vi "pco.labview_Live_Example_PSEUDO_COL.vi"() -> ()   [LabVIEW 2020]
doc: "A short program to demonstrate the fundamentals of control and image acquision with the pco.camera series. The program records a sequence of images, with \"live\" updating, until the \"StopRecording\" button is pressed. Use ctrl-H for more help on the individual controls and indicators.\n\nCopyright 2004, 2010 The Cooke Corporation."
uses:
  CameraAccess.lvlib
  ImageSensor.lvlib
  TimingControl.lvlib
  Recorder.lvlib
  RecordingControl.lvlib
  CameraDescription.lvlib
  Convert.lvlib
  GeneralCameraControl.lvlib
panel:
  in  "Auto Range Peak":bool
  in  "Auto Range Crop":bool
  in  "Load LUT":path
  in  "Gamma":dbl=1.0 min=0.009999999776482582 max=10.0 step=0.009999999776482582 format="%.2f"
  in  "iContrast [%]":i32 min=-100 max=100 step=1
  out "wImgBuf":u16[][](array[numeric])
  in  "Zoom [%]":i32(c297)=26
  in  "iScale_max":i32=2000 min=0 max=65535 step=1
  in  "iScale_min":i32=200 min=0 max=65535 step=1
  out "phConv":u64
  out "Image":picture
  out "Recorded Images":u32
  in  "TriggerMode":u16(ring) items=["auto sequence"=0, "software trigger"=1, "external exposure start & software trigger"=2, "external exposure control"=3, "external synchronized"=4, "fast external exposure control"=5, "external CDS control"=6, "slow external exposure control"=7, "external synchronized HDSDI"=258]
  in  "Quit":bool
  out "Error":errorcluster {"code" format="%x"}
  in  "Stop Record":bool
  out "Recording On":bool
  in  "roiY1":u16=2 min=2 max=2160 step=1
  in  "roiX1":u16=2 min=2 max=2560 step=1
  in  "roiY0":u16=1 min=1 max=2159 step=1
  in  "roiX0":u16=1 min=1 max=2559 step=1
  out "Image Height":u16
  out "Image Width":u16
  in  "Image Index":u32 max=9
  in  "dwImgCount":u32=10 caption="Required Number of Images" min=4 max=1565
  in  "DelayTimeBase":u16(ring)=2 items=["nanoseconds", "microseconds", "milliseconds"]
  in  "ExposureTimeBase":u16(ring)=2 items=["nanoseconds", "microseconds", "milliseconds"]
  in  "Exposure":u32=10 min=1
  in  "Delay":u32
  in  "Rate":i32(ring) items=["Low", "High"]
  # "This example is only suitable for monochrome cameras\n\nThis example is similar to pco.labview_Live_Example.vi, but suited for pseudo color conversion of bw cameras.\nBecause in addition here also the convert library is used in order to get a scaled and pseudo colored image that is displayed\nIt is possible to load any LUT that fits to the 4 possible formats, \nthe image value range can be selected with iScale_min/iScale_max, additionally contrast and gamma values can be selected\n\nUsage:\nSelect your required image count and the camera setup before you start the program.\nOnce started, the camera will be opened, the recorder will be created, initialized and images will be recorded and displayed automatically\nYou can stop the images by pressing stop record.\nAfter stopped, the image at the selected index will be read out\nTo finish the program click on quit application, this will force free and delete of the recorder and a close camera\nYou can change your required ROI, the value range, scaling, gamma, contrast and LUT after and also during record."
  # "pco.labview"
  # "Camera Setup"
  # "Recording Control"
  # "Parameters for image readout"
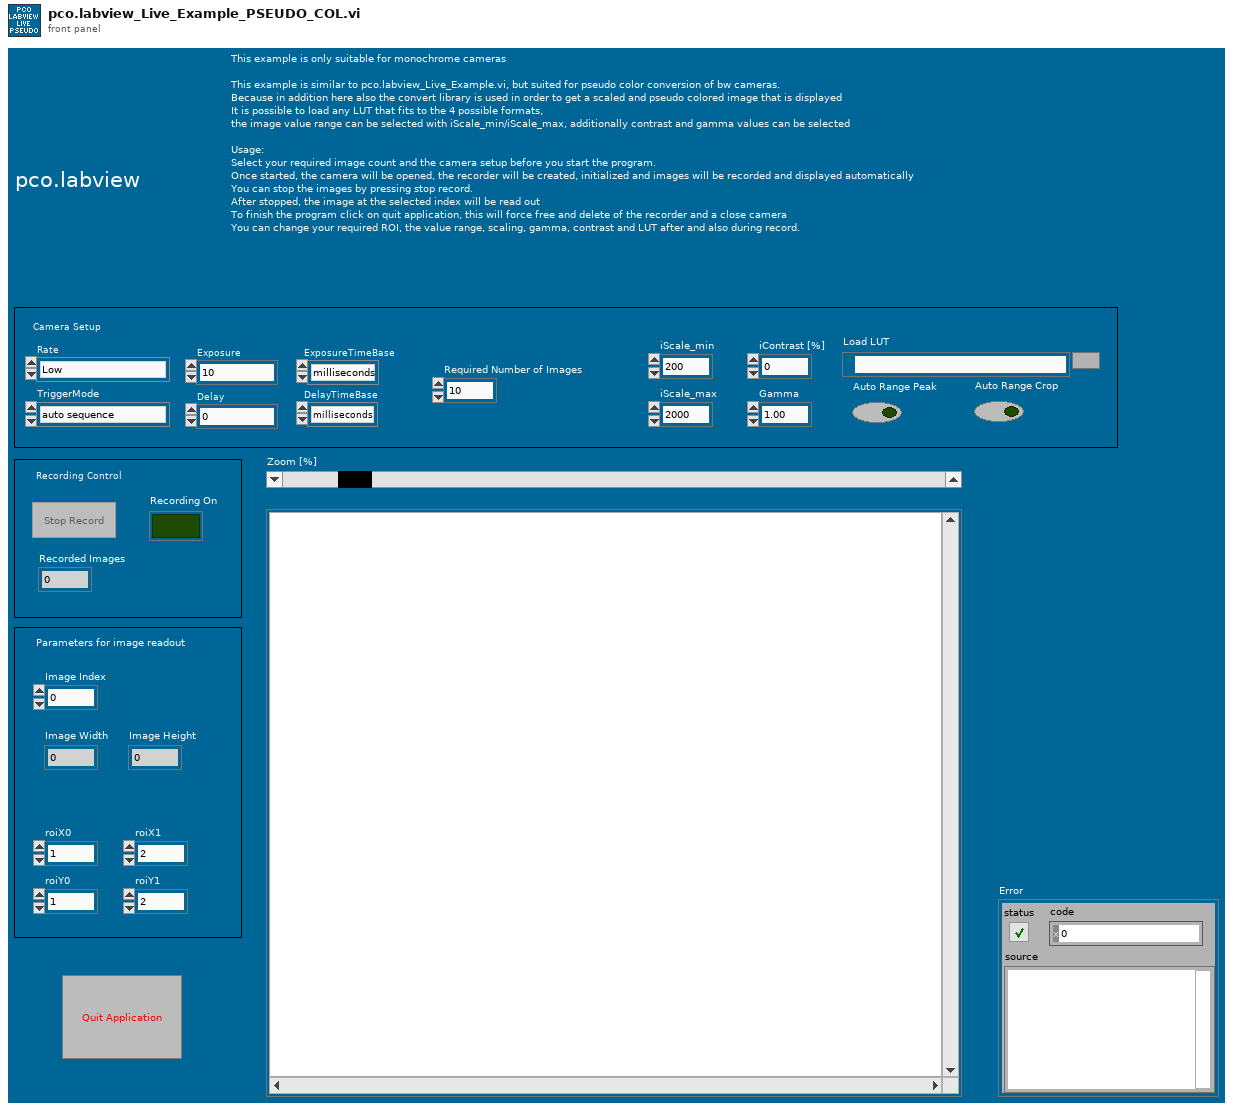
[diagram p1: front panel]
types:
  T1 = enum8{"Enabled", "Disabled", "Disabled and Grayed Out"}
  T2 = cluster{"wSensorTypeDESC":u16, "wSensorSubTypeDESC":u16, "wMaxHorzResStdDESC":u16, "wMaxVertResStdDESC":u16, "wMaxHorzResExtDESC":u16, "wMaxVertResExtDESC":u16, "wDynResDESC":u16, "wMaxBinHorzDESC":u16, "wBinHorzSteppingDESC":u16, "wMaxBinVertDESC":u16, "wBinVertSteppingDESC":u16, "wRoiHorStepsDESC":u16, "wRoiVertStepsDESC":u16, "wNumADCsDESC":u16, "wMinSizeHorzDESC":u16, "dwPixelRateDESC":u32[], "wConvFactDESC":u16[], "sCoolingSetpoints":i16[], "wSoftRoiHorStepsDESC":u16, "wSoftRoiVertStepsDESC":u16, "wIRDESC":u16, "wMinSizeVertDESC":u16, "dwMinDelayDESC":u32, "dwMaxDelayDESC":u32, "dwMinDelayStepDESC":u32, "dwMinExposureDESC":u32, "dwMaxExposureDESC":u32, "dwMinExposureStepDESC":u32, "dwMinDelayIRDESC":u32, "dwMaxDelayIRDESC":u32, "dwMinExposureIRDESC":u32, "dwMaxExposureIRDESC":u32, "wTimeTableDESC":u16, "wDoubleImageDESC":u16, "sMinCoolSetDESC":i16, "sMaxCoolSetDESC":i16, "sDefaultCoolSetDESC":i16, "wPowerDownModeDESC":u16, "wOffsetRegulationDESC":u16, "wColorPatternDESC":u16, "wPatternTypeDESC":u16, "wNumCoolingSetpoints":u16, "dwGeneralCapsDESC1":u32, "dwGeneralCapsDESC2":u32, "dwExtSyncFrequency":u32[], "dwGeneralCapsDESC3":u32, "dwGeneralCapsDESC4":u32}
  T3 = cluster{"wScale_minmax":u16, "iScale_maxmax":i32, "iScale_min":i32, "iScale_max":i32, "iColor_temp":i32, "iColor_tint":i32, "iColor_saturation":i32, "iColor_vibrance":i32, "iContrast":i32, "iGamma":i32, "iSRGB":i32, "pHistogramData":u64, "dwProcessingFlags":u32, "wProzValue4Min":u16, "wProzValue4Max":u16}
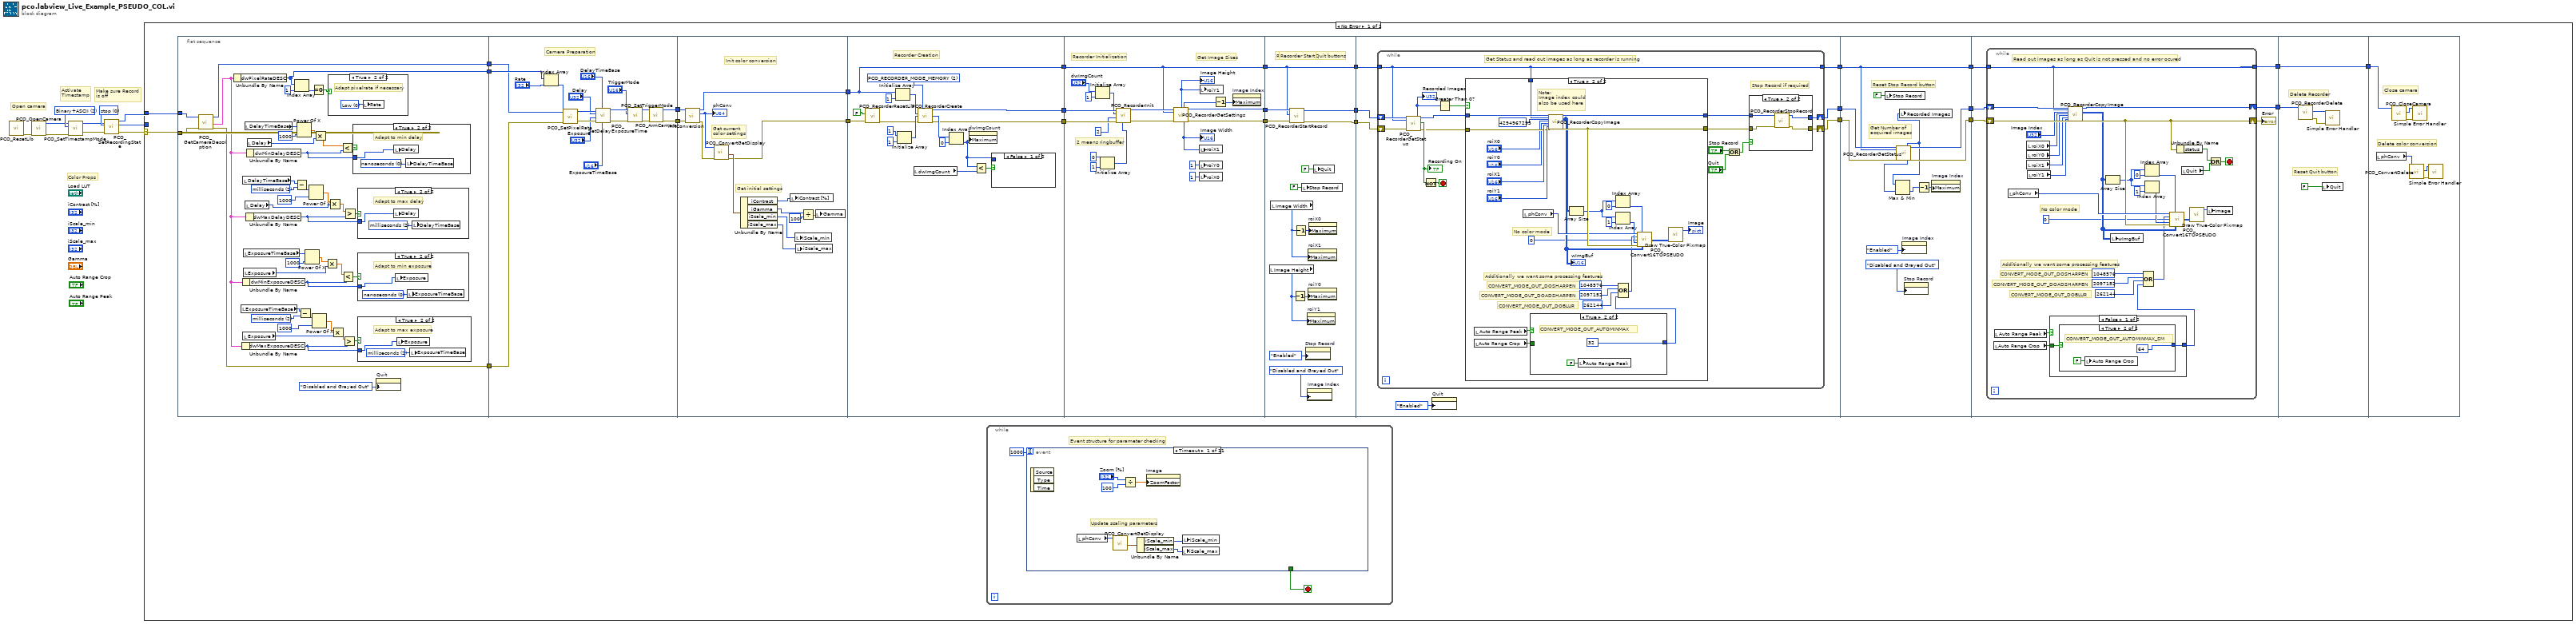
[diagram p0: block diagram]
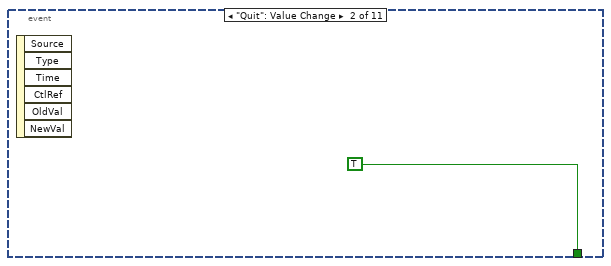
[diagram p2: hidden frame]
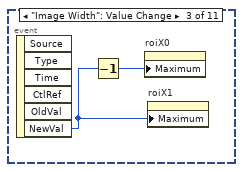
[diagram p3: hidden frame]
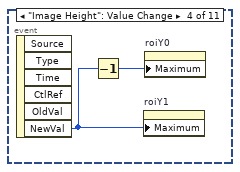
[diagram p4: hidden frame]
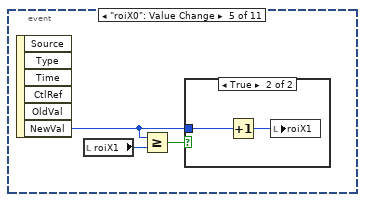
[diagram p5: hidden frame]
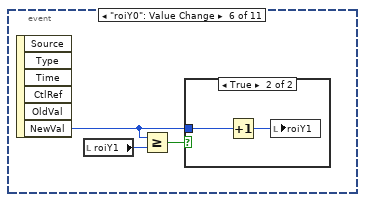
[diagram p7: hidden frame]
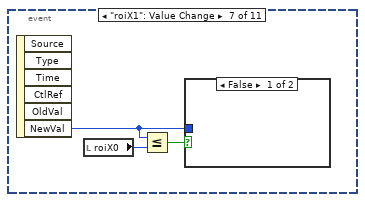
[diagram p9: hidden frame]
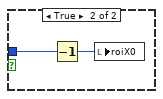
[diagram p10: hidden frame]
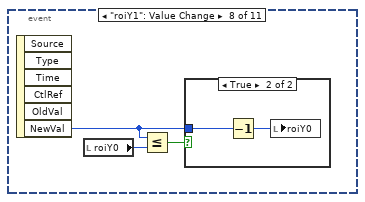
[diagram p11: hidden frame]
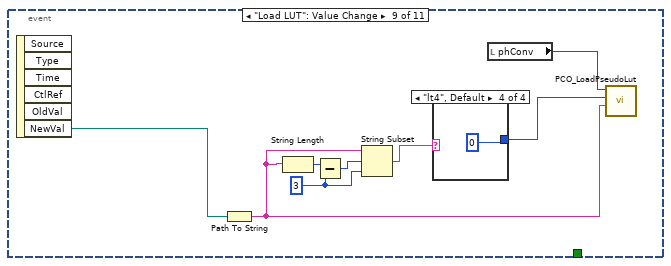
[diagram p13: hidden frame]
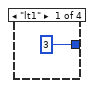
[diagram p14: hidden frame]
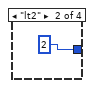
[diagram p15: hidden frame]
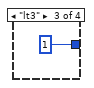
[diagram p16: hidden frame]
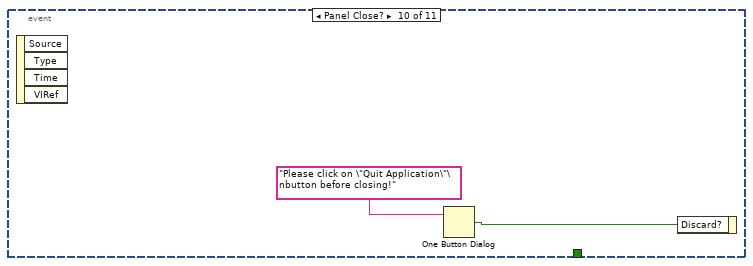
[diagram p17: hidden frame]
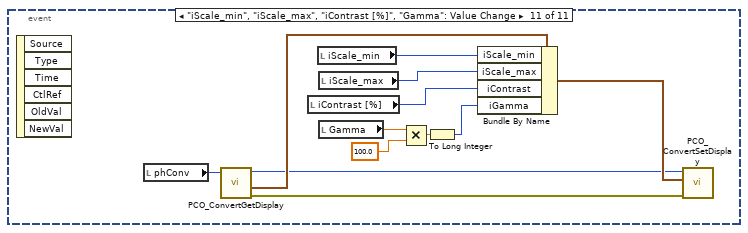
[diagram p18: hidden frame]
diagram:
  w3 = u16 2 items=["OFF", "Binary", "Binary+ASCII", "ASCII"] ("wTimeStampMode")
  w9 = u16 0 items=["stop", "run"] ("wRecState")
  # "Color Props"
  # "Activate\nTimestamp"
  # "Make sure Record \nis off"
  # "Open camera"
  n1 = call "PCO_ResetLib.vi"() -> ("error out"=w10:errorcluster)  [unwired: 10 in, 1 out]
  n2 = call "PCO_OpenCamera.vi"("error in (no error)"=w10) -> ("error out"=w1:errorcluster, "ph out"=w2:u64)  [unwired: 8 in, 1 out]
  n3 = call "PCO_SetTimestampMode.vi"("error in (no error)"=w1, "wTimeStampMode"=w3, "ph"=w2) -> ("error out"=w4:errorcluster, "ph out"=w5:u64)  [unwired: 6 in, 1 out]
  n4 = call "PCO_SetRecordingState.vi"("error in (no error)"=w4, "wRecState"=w9, "ph"=w5) -> ("error out"=w7:errorcluster, "ErrorMessage"=w6:i32, "ph out"=w8:u64)  [unwired: 6 in]
  n5 = case shown="No Error" w7 {
    selector: w7 -> [w36 w363]
    tunnel: w8 -> [w37 _]
    tunnel: w6 -> [_ w362]
    frame No Error {
      n6 = flat-sequence {
        tunnel: w36 -> [w136]
        tunnel: w37 -> [w137]
        tunnel: [w132] -> w20
        tunnel: [w139] -> w19
        tunnel: [w138] -> w18
        tunnel: [w152] -> w14
        tunnel: w20 -> [w155]
        tunnel: w19 -> [w149]
        tunnel: w18 -> [w150]
        tunnel: [w151] -> w11
        tunnel: w14 -> [w173]
        tunnel: [w170] -> w13
        tunnel: [w171] -> w12
        tunnel: w11 -> [w172]
        tunnel: w13 -> [w195]
        tunnel: w12 -> [w184]
        tunnel: [w186] -> w35
        tunnel: [w185] -> w34
        tunnel: [w184] -> w31
        tunnel: w35 -> [w217]
        tunnel: w34 -> [w216]
        tunnel: [w207] -> w33
        tunnel: [w208] -> w32
        tunnel: w31 -> [w206]
        tunnel: [w206] -> w30
        tunnel: w33 -> [w228]
        tunnel: w32 -> [w227]
        tunnel: w30 -> [w226]
        tunnel: [w226] -> w17
        tunnel: [w221] -> w16
        tunnel: [w220] -> w15
        tunnel: w17 -> [w237]
        tunnel: [w234] -> w28
        tunnel: [w233] -> w26
        tunnel: [w235] -> w24
        tunnel: w16 -> [w232]
        tunnel: w15 -> [w231]
        tunnel: [w303] -> w29
        tunnel: w28 -> [w305]
        tunnel: [w302] -> w27
        tunnel: w26 -> [w306]
        tunnel: [w304] -> w25
        tunnel: w24 -> [w304]
        tunnel: w29 -> [w313]
        tunnel: w27 -> [w312]
        tunnel: w25 -> [w311]
        tunnel: [w309] -> w23
        tunnel: [w308] -> w22
        tunnel: w23 -> [w354]
        tunnel: w22 -> [w351]
        tunnel: [w351] -> w21
        tunnel: w21 -> [w361]
        frame #0 {
          w99 = u16 2 items=["nanoseconds", "microseconds", "milliseconds"] ("DelayTimeBase")
          w102 = u16 2 items=["nanoseconds", "microseconds", "milliseconds"] ("DelayTimeBase")
          n7 = call "PCO_GetCameraDescription.vi"("error in (no error)"=w136, "ph"=w137) -> ("error out"=w139:errorcluster, "strDescription"=w98:T2, "ph out"=w138:u64)  [unwired: 6 in, 1 out]
          n8 = Unbundle By Name(w98) -> ("dwPixelRateDESC"=w132:u32[])
          n9 = local read "ExposureTimeBase"() -> (w100:u16)
          n10 = Unbundle By Name(w98) -> ("dwMaxExposureDESC"=w129:u32)
          n11 = Unbundle By Name(w98) -> ("dwMinExposureDESC"=w128:u32)
          n12 = local read "DelayTimeBase"() -> (w101:u16)
          n13 = local read "Exposure"() -> (w107:u32)
          n14 = local read "ExposureTimeBase"() -> (w120:u16)
          n15 = local read "Exposure"() -> (w105:u32)
          n16 = local read "DelayTimeBase"() -> (w127:u16)
          n17 = local read "Delay"() -> (w112:u32)
          n18 = Unbundle By Name(w98) -> ("dwMaxDelayDESC"=w130:u32)
          n19 = Unbundle By Name(w98) -> ("dwMinDelayDESC"=w125:u32)
          n20 = local read "Delay"() -> (w123:u32)
          n21 = Index Array(array=w132, index=1) -> (element=w134:u32)
          n22 = Subtract(x=w101, y=w102) -> (x-y=w116:i32)
          n23 = Power Of X(1:u32 1000 ("Delay"), 2:w127) -> (0:w124:dbl)
          n24 = Subtract(x=w100, y=w99) -> (x-y=w108:i32)
          n25 = Power Of X(1:u32 1000 ("Delay"), 2:w120) -> (0:w119:dbl)
          n26 = Power Of X(1:u32 1000 ("Delay"), 2:w116) -> (0:w113:dbl)
          n27 = Equal To 0?(x=w134) -> (x = 0?=w133:bool)
          n28 = Power Of X(1:u32 1000 ("Delay"), 2:w108) -> (0:w110:dbl)
          n29 = Multiply(x=w124, y=w123) -> (x*y=w122:dbl)
          n30 = Multiply(x=w119, y=w105) -> (x*y=w104:dbl)
          n31 = Multiply(x=w113, y=w112) -> (x*y=w114:dbl)
          n32 = case shown="True" w133 {
            frame False {
            }
            frame True {
              w148 = 0 items=["Low", "High"] ("Rate")
              # "Adapt pixelrate if necessary"
              n33 = local write "Rate"(w148) -> ()
            }
          }
          n34 = Multiply(x=w110, y=w107) -> (x*y=w106:dbl)
          n35 = Less?(x=w122, y=w125) -> (x < y?=w121:bool)
          n36 = Less?(x=w104, y=w128) -> (x < y?=w103:bool)
          n37 = Greater?(x=w106, y=w129) -> (0:w111:bool)
          n38 = Greater?(x=w114, y=w130) -> (0:w117:bool)
          n39 = case shown="True" w121 {
            tunnel: w125 -> [_ w147]
            frame False {
            }
            frame True {
              w146 = u16 0 items=["nanoseconds", "microseconds", "milliseconds"] ("DelayTimeBase")
              # "Adapt to min delay"
              n40 = local write "Delay"(w147) -> ()
              n41 = local write "DelayTimeBase"(w146) -> ()
            }
          }
          n42 = case shown="True" w117 {
            tunnel: w130 -> [_ w145]
            frame False {
            }
            frame True {
              w144 = u16 2 items=["nanoseconds", "microseconds", "milliseconds"] ("DelayTimeBase")
              # "Adapt to max delay"
              n43 = local write "Delay"(w145) -> ()
              n44 = local write "DelayTimeBase"(w144) -> ()
            }
          }
          n45 = case shown="True" w103 {
            tunnel: w128 -> [_ w143]
            frame False {
            }
            frame True {
              w142 = u16 0 items=["nanoseconds", "microseconds", "milliseconds"] ("DelayTimeBase")
              # "Adapt to min exposure"
              n46 = local write "Exposure"(w143) -> ()
              n47 = local write "ExposureTimeBase"(w142) -> ()
            }
          }
          n48 = case shown="True" w111 {
            tunnel: w129 -> [_ w141]
            frame False {
            }
            frame True {
              w140 = u16 2 items=["nanoseconds", "microseconds", "milliseconds"] ("DelayTimeBase")
              # "Adapt to max exposure"
              n49 = local write "Exposure"(w141) -> ()
              n50 = local write "ExposureTimeBase"(w140) -> ()
            }
          }
          n51 = property on="Quit" class="Bool (strict)"("DisabledEnum"=T1."Disabled and Grayed Out" ("Disabled")) -> ()  [unwired: 2 in, 2 out]
        }
        frame #1 {
          # "Camera Preparation"
          n52 = Index Array(array=w155, index="Rate") -> (element=w165:u32)
          n53 = call "PCO_SetPixelRate.vi"("error in (no error)"=w149, "dwPixelRate"=w165, "ph"=w150) -> ("error out"=w163:errorcluster, "ph out"=w164:u64)  [unwired: 6 in, 1 out]
          n54 = call "PCO_SetDelayExposureTime.vi"("wTimeBaseExposure"="ExposureTimeBase", "wTimeBaseDelay"="DelayTimeBase", "error in (no error)"=w163, "dwExposure"="Exposure", "dwDelay"="Delay", "ph"=w164) -> ("error out"=w157:errorcluster, "ph out"=w158:u64)  [unwired: 3 in, 1 out]
          n55 = call "PCO_SetTriggerMode.vi"("error in (no error)"=w157, "wTriggerMode"="TriggerMode", "ph"=w158) -> ("error out"=w153:errorcluster, "ph out"=w154:u64)  [unwired: 6 in, 1 out]
          n56 = call "PCO_ArmCamera.vi"("error in (no error)"=w153, "ph"=w154) -> ("error out"=w152:errorcluster, "ph out"=w151:u64)  [unwired: 7 in, 1 out]
        }
        frame #2 {
          # "Get initial settings"
          # "Get current\ncolor settings"
          # "Init color conversion"
          n57 = call "initConversion.vi"("phCam"=w172, "error in (no error)"=w173) -> ("ph out"=w171:u64, "phConv"=w176:u64, "error out"=w175:errorcluster)  [unwired: 8 in, 3 out]
          "phConv" <- w176
          n58 = call "PCO_ConvertGetDisplay.vi"("error in (no error)"=w175, "ph"=w176) -> ("error out"=w170:errorcluster, "strDisplay"=w174:T3)  [unwired: 6 in, 2 out]
          n59 = Unbundle By Name(w174) -> ("iContrast"=w177:i32, "iGamma"=w169:i32, "iScale_min"=w178:i32, "iScale_max"=w179:i32)
          n60 = local write "iContrast [%]"(w177) -> ()
          n61 = local write "iScale_min"(w178) -> ()
          n62 = local write "iScale_max"(w179) -> ()
          n63 = Divide(x=w169, y=100) -> (x/y=w168:dbl)
          n64 = local write "Gamma"(w168) -> ()
        }
        frame #3 {
          w180 = u16 2 items=["PCO_RECORDER_MODE_FILE"=1, "PCO_RECORDER_MODE_MEMORY"=2, "PCO_RECORDER_MODE_CAMRAM"=3] ("dwRecMode")
          # "Recorder Creation"
          n65 = call "PCO_RecorderResetLib.vi"("error in (no error)"=w195, "bSilent"=FALSE) -> ("error out"=w187:errorcluster)  [unwired: 8 in, 1 out]
          n66 = Initialize Array(w184, 1 ("dimension size")) -> (w193:u64[])
          n67 = Initialize Array(u32 1 ("dimension size"), 1 ("dimension size")) -> (w190:u32[])
          n68 = local read "dwImgCount"() -> (w181:u32)
          n69 = call "PCO_RecorderCreate.vi"("wRecMode"=w180, "phCamArr"=w193, "dwImgDistributionArr"=w190, "error in (no error)"=w187) -> ("phRec out"=w185:u64, "dwMaxImgCountArr"=w189:u32[], "error out"=w186:errorcluster)  [unwired: 8 in, 1 out]
          n70 = Index Array(array=w189, index=0) -> (element=w182:u32)
          n71 = property on="dwImgCount" class="DigNum (strict)"("Maximum"=w182) -> ()  [unwired: 2 in, 2 out]
          n72 = Less?(x=w182, y=w181) -> (x < y?=w183:bool)
          n73 = case shown="False" w183 {
            tunnel: w182 -> [_ w197]
            frame False {
            }
            frame True {
              n74 = local write "dwImgCount"(w197) -> ()
            }
          }
        }
        frame #4 {
          # "2 means ringbuffer"
          # "Get Image Sizes"
          # "Recorder Initialization"
          n75 = Initialize Array("dwImgCount", 1 ("dimension size")) -> (w213:u32[])
          n76 = Initialize Array(u16 0 ("element"), 1 ("dimension size")) -> (w198:u16[])
          n77 = call "PCO_RecorderInit.vi"("wRamSegmentArr"=w198, "error in (no error)"=w217, "wType"=u16 2, "dwImgCountArr"=w213, "phRec"=w216) -> ("error out"=w212:errorcluster, "phRec out"=w211:u64)  [unwired: 4 in, 1 out]
          n78 = call "PCO_RecorderGetSettings.vi"("phRec"=w211, "phCam"=w206, "error in (no error)"=w212) -> ("wHeight"=w205:u16, "dwReqImgCount"=w202:u32, "phRec out"=w207:u64, "wWidth"=w204:u16, "error out"=w208:errorcluster)  [unwired: 4 in, 4 out]
          "Image Height" <- w205
          "Image Width" <- w204
          n79 = local write "roiX1"(w204) -> ()
          n80 = local write "roiY0"(u16 1 ("roiY0")) -> ()
          n81 = local write "roiX0"(u16 1 ("roiY0")) -> ()
          n82 = local write "roiY1"(w205) -> ()
          n83 = Decrement(x=w202) -> (x-1=w203:u32)
          n84 = property on="Image Index" class="DigNum (strict)"("Maximum"=w203) -> ()  [unwired: 2 in, 2 out]
        }
        frame #5 {
          # "Reset Stop and Quit buttons"
          # "Recorder Start"
          n85 = local read "Image Height"() -> (w223:u16)
          n86 = local read "Image Width"() -> (w222:u16)
          n87 = call "PCO_RecorderStartRecord.vi"("error in (no error)"=w227, "phCam"=w226, "phRec"=w228) -> ("error out"=w220:errorcluster, "phRec out"=w221:u64)  [unwired: 6 in, 1 out]
          n88 = Decrement(x=w223) -> (x-1=w224:u16)
          n89 = Decrement(x=w222) -> (x-1=w225:u16)
          n90 = local write "Stop Record"(FALSE ("Stop Record")) -> ()
          n91 = property on="Stop Record" class="Bool (strict)"("DisabledEnum"=T1."Enabled" ("Disabled")) -> ()  [unwired: 2 in, 2 out]
          n92 = property on="roiY1" class="DigNum (strict)"("Maximum"=w223) -> ()  [unwired: 2 in, 2 out]
          n93 = property on="Image Index" class="DigNum (strict)"("DisabledEnum"=T1."Disabled and Grayed Out" ("Disabled")) -> ()  [unwired: 2 in, 2 out]
          n94 = property on="roiX1" class="DigNum (strict)"("Maximum"=w222) -> ()  [unwired: 2 in, 2 out]
          n95 = property on="roiY0" class="DigNum (strict)"("Maximum"=w224) -> ()  [unwired: 2 in, 2 out]
          n96 = property on="roiX0" class="DigNum (strict)"("Maximum"=w225) -> ()  [unwired: 2 in, 2 out]
          n97 = local write "Quit"(FALSE ("Stop")) -> ()
        }
        frame #6 {
          n98 = while {
            tunnel: w237 -> [w241]
            shift-right: [w245] -> w233
            shift-left: w231 -> [w253]
            shift-right: [w246] -> w234
            shift-left: w232 -> [w249]
            tunnel: [w241] -> w235
            stop <- w248 stop-if-true
            # "Stop Record if required"
            # "Get Status and read out images as long as recorder is running"
            n99 = call "PCO_RecorderGetStatus.vi"("phRec"=w249, "phCam"=w241, "error in (no error)"=w253) -> ("dwProcImgCount"=w238:u32, "phRec out"=w251:u64, "bIsRunning"=w252:bool, "error out"=w250:errorcluster)  [unwired: 5 in, 8 out]
            "Recording On" <- w252
            "Recorded Images" <- w238
            n100 = Not(x=w252) -> (.not. x?=w248:bool)
            n101 = Greater Than 0?(x=w238) -> (x > 0?=w239:bool)
            n102 = case shown="True" w239 {
              tunnel: w251 -> [w255 w282]
              tunnel: w250 -> [w254 w278]
              tunnel: [w255 w277] -> w242
              tunnel: w241 -> [_ w275]
              tunnel: [w254 w273] -> w240
              frame False {
              }
              frame True {
                # "No color mode"
                # "CONVERT_MODE_OUT_DOBLUR"
                # "CONVERT_MODE_OUT_DOADSHARPEN"
                # "CONVERT_MODE_OUT_DOSHARPEN"
                # "Additionally we want some processing features"
                # "Note: \nImage index could \nalso be used here"
                n103 = local read "Auto Range Crop"() -> (w257:bool)
                n104 = local read "Auto Range Peak"() -> (w258:bool)
                n105 = local read "phConv"() -> (w272:u64)
                n106 = case shown="True" w258 {
                  tunnel: [w283 32 ("colorMode")] -> w256
                  tunnel: w257 -> [w284 _]
                  frame False {
                    n107 = case shown="False" w284 {
                      tunnel: [0 ("colorMode") 64 ("colorMode")] -> w283
                      frame False {
                      }
                      frame True {
                        # "CONVERT_MODE_OUT_AUTOMINMAX_SM"
                        n108 = local write "Auto Range Crop"(FALSE ("Auto Range Crop")) -> ()
                      }
                    }
                  }
                  frame True {
                    # "CONVERT_MODE_OUT_AUTOMINMAX"
                    n109 = local write "Auto Range Peak"(FALSE ("Auto Range Peak")) -> ()
                  }
                }
                n110 = call "PCO_RecorderCopyImage.vi"("phRec"=w282, "phCam"=w275, "dwImgIdx"=u32 4294967295, "wRoiX0"="roiX0", "wRoiY0"="roiY0", "wRoiX1"="roiX1", "wRoiY1"="roiY1", "error in (no error)"=w278) -> ("phRec out"=w277:u64, "wImgBuf"=w271:u16[][], "error out"=w273:errorcluster)  [unwired: 13 in, 4 out]
                "wImgBuf" <- w271
                n111 = Array Size(array=w271) -> (size(s)=w267:i32[])
                n112 = Index Array(array=w267, index=0) -> (element=w269:i32)
                n113 = Index Array(array=w267, index=1) -> (element=w266:i32)
                n114 = Compound Arithmetic op=OR ("Mehrfacharithmetik")(1048576 ("colorMode"), 2097152 ("colorMode"), 262144 ("colorMode"), w256) -> (w260:i32)
                n115 = call "PCO_Convert16TOPSEUDO.vi"("ph"=w272, "height"=w269, "mode"=w260, "icolmode"=0 ("mode"), "width"=w266, "error in (no error)"=w273, "b16"=w271) -> ("b32"=w274:u32[][])  [unwired: 5 in, 3 out]
                n116 = call "Draw True-Color Pixmap.vi"("data (RGB format)"=w274) -> ("new picture"=→"Image":picture)  [unwired: 8 in]
              }
            }
            n117 = Or(x="Stop Record", y="Quit") -> (x .or. y?=w247:bool)
            n118 = case shown="True" w247 {
              tunnel: w242 -> [w291 w295]
              tunnel: w240 -> [w290 w294]
              tunnel: [w291 w292] -> w246
              tunnel: [w290 w293] -> w245
              frame False {
              }
              frame True {
                n119 = call "PCO_RecorderStopRecord.vi"("error in (no error)"=w294, "phRec"=w295) -> ("error out"=w293:errorcluster, "phRec out"=w292:u64)  [unwired: 7 in, 1 out]
              }
            }
          }
          n120 = property on="Quit" class="Bool (strict)"("DisabledEnum"=T1."Enabled" ("Disabled")) -> ()  [unwired: 2 in, 2 out]
        }
        frame #7 {
          # "Get Number of \nacquired images"
          # "Reset Stop Record button"
          n121 = local write "Stop Record"(FALSE ("Stop Record")) -> ()
          n122 = call "PCO_RecorderGetStatus.vi"("phRec"=w305, "phCam"=w304, "error in (no error)"=w306) -> ("dwProcImgCount"=w299:u32, "dwReqImgCount"=w298:u32, "phRec out"=w303:u64, "error out"=w302:errorcluster)  [unwired: 5 in, 8 out]
          n123 = Max & Min(x=w299, y=w298) -> (min(x,y)=w300:u32)  [unwired: 1 out]
          n124 = local write "Recorded Images"(w299) -> ()
          n125 = property on="Image Index" class="DigNum (strict)"("DisabledEnum"=T1."Enabled" ("Disabled")) -> ()  [unwired: 2 in, 2 out]
          n126 = property on="Stop Record" class="Bool (strict)"("DisabledEnum"=T1."Disabled and Grayed Out" ("Disabled")) -> ()  [unwired: 2 in, 2 out]
          n127 = Decrement(x=w300) -> (x-1=w301:u32)
          n128 = property on="Image Index" class="DigNum (strict)"("Maximum"=w301) -> ()  [unwired: 2 in, 2 out]
        }
        frame #8 {
          n129 = while {
            shift-right: [w330] -> w310
            shift-left: w312 -> [w340]
            shift-right: [w334] -> w309
            shift-left: w313 -> [w339]
            tunnel: w311 -> [w333]
            tunnel: [w333] -> w308
            stop <- w341 stop-if-true
            # "No color mode"
            # "CONVERT_MODE_OUT_DOBLUR"
            # "CONVERT_MODE_OUT_DOADSHARPEN"
            # "CONVERT_MODE_OUT_DOSHARPEN"
            # "Additionally we want some processing features"
            # "Read out images as long as Quit is not pressed and no error ocured"
            n130 = local read "Auto Range Crop"() -> (w316:bool)
            n131 = local read "Auto Range Peak"() -> (w315:bool)
            n132 = local read "phConv"() -> (w332:u64)
            n133 = local read "roiX0"() -> (w324:u16)
            n134 = local read "roiY0"() -> (w323:u16)
            n135 = local read "roiX1"() -> (w337:u16)
            n136 = local read "roiY1"() -> (w336:u16)
            n137 = case shown="False" w315 {
              tunnel: [w344 32 ("colorMode")] -> w314
              tunnel: w316 -> [w345 _]
              frame False {
                n138 = case shown="True" w345 {
                  tunnel: [0 ("colorMode") 64 ("colorMode")] -> w344
                  frame False {
                  }
                  frame True {
                    # "CONVERT_MODE_OUT_AUTOMINMAX_SM"
                    n139 = local write "Auto Range Crop"(FALSE ("Auto Range Crop")) -> ()
                  }
                }
              }
              frame True {
                # "CONVERT_MODE_OUT_AUTOMINMAX"
                n140 = local write "Auto Range Peak"(FALSE ("Auto Range Peak")) -> ()
              }
            }
            n141 = call "PCO_RecorderCopyImage.vi"("phRec"=w339, "phCam"=w333, "dwImgIdx"="Image Index", "wRoiX0"=w324, "wRoiY0"=w323, "wRoiX1"=w337, "wRoiY1"=w336, "error in (no error)"=w340) -> ("phRec out"=w334:u64, "wImgBuf"=w322:u16[][], "error out"=w330:errorcluster)  [unwired: 13 in, 4 out]
            n142 = Array Size(array=w322) -> (size(s)=w327:i32[])
            n143 = local write "wImgBuf"(w322) -> ()
            n144 = Compound Arithmetic op=OR ("Mehrfacharithmetik")(1048576 ("colorMode"), 2097152 ("colorMode"), 262144 ("colorMode"), w314) -> (w317:i32)
            n145 = Index Array(array=w327, index=0) -> (element=w326:i32)
            n146 = Index Array(array=w327, index=1) -> (element=w325:i32)
            n147 = call "PCO_Convert16TOPSEUDO.vi"("ph"=w332, "height"=w326, "mode"=w317, "icolmode"=0 ("mode"), "width"=w325, "error in (no error)"=w330, "b16"=w322) -> ("b32"=w331:u32[][])  [unwired: 5 in, 3 out]
            n148 = Unbundle By Name(w330) -> ("status"=w343:bool)
            n149 = local read "Quit"() -> (w342:bool)
            n150 = call "Draw True-Color Pixmap.vi"("data (RGB format)"=w331) -> ("new picture"=w335:picture)  [unwired: 8 in]
            n151 = local write "Image"(w335) -> ()
            n152 = Or(x=w343, y=w342) -> (x .or. y?=w341:bool)
          }
          "Error" <- w310
        }
        frame #9 {
          # "Delete Recorder"
          # "Reset Quit button"
          n153 = call "PCO_RecorderDelete.vi"("phRec"=w354) -> ("error out"=w352:errorcluster, "ErrorMessage"=w353:i32)  [unwired: 9 in]
          n154 = local write "Quit"(FALSE ("Stop Record")) -> ()
          n155 = call "Simple Error Handler.vi"("error code (no error:0)"=w353, "error in (no error)"=w352) -> ()  [unwired: 3 in, 5 out]
        }
        frame #10 {
          # "Delete color conversion"
          # "Close camera"
          n156 = local read "phConv"() -> (w358:u64)
          n157 = call "PCO_CloseCamera.vi"("ph"=w361) -> ("error out"=w359:errorcluster, "ErrorMessage"=w360:i32)  [unwired: 9 in]
          n158 = call "PCO_ConvertDelete.vi"("ph"=w358) -> ("error out"=w356:errorcluster, "ErrorMessage"=w357:i32)  [unwired: 9 in]
          n159 = call "Simple Error Handler.vi"("error code (no error:0)"=w360, "error in (no error)"=w359) -> ()  [unwired: 3 in, 5 out]
          n160 = call "Simple Error Handler.vi"("error code (no error:0)"=w357, "error in (no error)"=w356) -> ()  [unwired: 3 in, 5 out]
        }
      }
      n161 = while {
        stop <- w38 stop-if-true
        # "Event structure for parameter checking"
        n162 = event shown="[0] Timeout" {
          selector: _ -> [_ _ _ _ _ _ _ _ _ _ _]
          dyn-events: _ -> [_ _ _ _ _ _ _ _ _ _ _]
          timeout: 1000 -> [_ _ _ _ _ _ _ _ _ _ _]
          tunnel: [_ TRUE _ _ _ _ _ _ _ _ _] -> w38
          event Timeout {
            # "Update scaling parameters"
            n163 = event-data() -> ()  [unwired: 1 in, 3 out]
            n164 = local read "phConv"() -> (w43:u64)
            n165 = call "PCO_ConvertGetDisplay.vi"("ph"=w43) -> ("strDisplay"=w42:T3)  [unwired: 7 in, 3 out]
            n166 = Divide(x="Zoom [%]", y=100) -> (x/y=w44:dbl)
            n167 = Unbundle By Name(w42) -> ("iScale_min"=w40:i32, "iScale_max"=w41:i32)
            n168 = property on="Image" class="Pict"("ZoomFactor"=w44) -> ()  [unwired: 2 in, 2 out]
            n169 = local write "iScale_max"(w41) -> ()
            n170 = local write "iScale_min"(w40) -> ()
          }
          event "Quit": Value Change {
            n171 = event-data() -> ()  [unwired: 1 in, 6 out]
          }
          event "Image Width": Value Change {
            n172 = event-data() -> ("NewVal"=w48:u16)  [unwired: 1 in, 5 out]
            n173 = Decrement(x=w48) -> (x-1=w49:u16)
            n174 = property on="roiX0" class="DigNum (strict)"("Maximum"=w49) -> ()  [unwired: 2 in, 2 out]
            n175 = property on="roiX1" class="DigNum (strict)"("Maximum"=w48) -> ()  [unwired: 2 in, 2 out]
          }
          event "Image Height": Value Change {
            n176 = event-data() -> ("NewVal"=w50:u16)  [unwired: 1 in, 5 out]
            n177 = Decrement(x=w50) -> (x-1=w51:u16)
            n178 = property on="roiY1" class="DigNum (strict)"("Maximum"=w50) -> ()  [unwired: 2 in, 2 out]
            n179 = property on="roiY0" class="DigNum (strict)"("Maximum"=w51) -> ()  [unwired: 2 in, 2 out]
          }
          event "roiX0": Value Change {
            n180 = event-data() -> ("NewVal"=w52:u16)  [unwired: 1 in, 5 out]
            n181 = local read "roiX1"() -> (w54:u16)
            n182 = Greater Or Equal?(x=w52, y=w54) -> (x >= y?=w53:bool)
            n183 = case shown="True" w53 {
              tunnel: w52 -> [_ w56]
              frame False {
              }
              frame True {
                n184 = Increment(x=w56) -> (x+1=w55:u16)
                n185 = local write "roiX1"(w55) -> ()
              }
            }
          }
          event "roiY0": Value Change {
            n186 = event-data() -> ("NewVal"=w57:u16)  [unwired: 1 in, 5 out]
            n187 = local read "roiY1"() -> (w59:u16)
            n188 = Greater Or Equal?(x=w57, y=w59) -> (x >= y?=w58:bool)
            n189 = case shown="True" w58 {
              tunnel: w57 -> [_ w61]
              frame False {
              }
              frame True {
                n190 = Increment(x=w61) -> (x+1=w60:u16)
                n191 = local write "roiY1"(w60) -> ()
              }
            }
          }
          event "roiX1": Value Change {
            n192 = event-data() -> ("NewVal"=w62:u16)  [unwired: 1 in, 5 out]
            n193 = local read "roiX0"() -> (w64:u16)
            n194 = Less Or Equal?(x=w62, y=w64) -> (x <= y?=w63:bool)
            n195 = case shown="False" w63 {
              tunnel: w62 -> [_ w66]
              frame False {
              }
              frame True {
                n196 = Decrement(x=w66) -> (x-1=w65:u16)
                n197 = local write "roiX0"(w65) -> ()
              }
            }
          }
          event "roiY1": Value Change {
            n198 = event-data() -> ("NewVal"=w67:u16)  [unwired: 1 in, 5 out]
            n199 = local read "roiY0"() -> (w69:u16)
            n200 = Less Or Equal?(x=w67, y=w69) -> (x <= y?=w68:bool)
            n201 = case shown="True" w68 {
              tunnel: w67 -> [_ w71]
              frame False {
              }
              frame True {
                n202 = Decrement(x=w71) -> (x-1=w70:u16)
                n203 = local write "roiY0"(w70) -> ()
              }
            }
          }
          event "Load LUT": Value Change {
            w76 = 3 ("y")
            n204 = event-data() -> ("NewVal"=w72:path)  [unwired: 1 in, 5 out]
            n205 = Path To String(path=w72) -> (string=w73:string)
            n206 = String Length(string=w73) -> (length=w78:i32)
            n207 = Subtract(x=w78, y=w76) -> (x-y=w77:i32)
            n208 = String Subset(string=w73, offset (0)=w77, length (rest)=w76) -> (substring=w75:string)
            n209 = case shown="\"lt4\", Default" w75 {
              tunnel: [3 2 1 0] -> w74
              frame "lt1" {
              }
              frame "lt2" {
              }
              frame "lt3" {
              }
              frame "lt4", Default {
              }
            }
            n210 = local read "phConv"() -> (w79:u64)
            n211 = call "PCO_LoadPseudoLut.vi"("filename"=w73, "format"=w74, "ph"=w79) -> ()  [unwired: 6 in, 3 out]
          }
          event Panel Close? {
            n212 = event-data() -> ()  [unwired: 1 in, 4 out]
            n213 = One Button Dialog(message="Please click on \"Quit Application\"\nbutton before closing!") -> (true=w84:bool)  [unwired: 1 in]
            n214 = event-data("Discard?"=w84) -> ()  [unwired: 1 in, 1 out]
          }
          event "iScale_min", "iScale_max", "iContrast [%]", "Gamma": Value Change {
            n215 = event-data() -> ()  [unwired: 1 in, 6 out]
            n216 = local read "phConv"() -> (w97:u64)
            n217 = call "PCO_ConvertGetDisplay.vi"("ph"=w97) -> ("error out"=w90:errorcluster, "strDisplay"=w95:T3, "ph out"=w91:u64)  [unwired: 7 in, 1 out]
            n218 = local read "iContrast [%]"() -> (w92:i32)
            n219 = local read "iScale_min"() -> (w94:i32)
            n220 = local read "iScale_max"() -> (w93:i32)
            n221 = local read "Gamma"() -> (w89:dbl)
            n222 = Multiply(x=w89, y=100.0) -> (x*y=w87:dbl)
            n223 = To Long Integer(number=w87) -> (32bit integer=w86:i32)
            n224 = Bundle By Name(cluster=w95, "iScale_min"=w94, "iScale_max"=w93, "iContrast"=w92, "iGamma"=w86) -> (w96:T3)
            n225 = call "PCO_ConvertSetDisplay.vi"("error in (no error)"=w90, "strDisplay"=w96, "ph"=w91) -> ()  [unwired: 6 in, 3 out]
          }
        }
      }
    }
    frame Error {
      n226 = call "Simple Error Handler.vi"("error code (no error:0)"=w362, "error in (no error)"=w363) -> ()  [unwired: 3 in, 5 out]
    }
  }
